vi "Tests Folder.vi"(3 "Relative Path (\"\" - Folder)":string) -> (1 "Tests Folder":path)   [LabVIEW 2011]
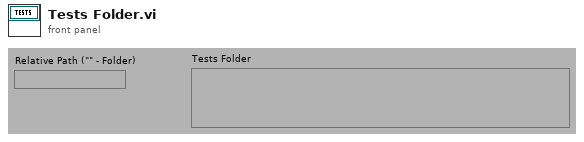
[diagram p1: front panel]
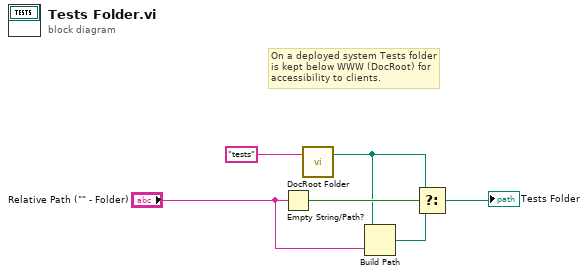
[diagram p0: block diagram]
diagram:
  # "On a deployed system Tests folder\nis kept below WWW (DocRoot) for\naccessibility to clients."
  n1 = Empty String/Path?(string/path="Relative Path (\"\" - Folder)") -> (empty?=w5:bool)
  n2 = call "DocRoot Folder.vi"("Relative Path (\"\" - Folder)"="tests" ("name or relative path")) -> ("DocumentRoot Folder"=w1:path)  [unwired: 2 in]
  n3 = Build Path(base path=w1, name or relative path="Relative Path (\"\" - Folder)") -> (appended path=w3:path)
  n4 = Select(t=w1, s=w5, f=w3) -> (s? t:f=→"Tests Folder":path)
